vi "data表转mysql表.vi"(11 "data":string[](array[string])) -> (3 "mysqldata簇":T1 {"JCSJ" format="%<%Y/%m/%d %H:%M:%S>T"})   [LabVIEW 2016]
panel:
  out "mysql完整簇":T2 {"JCSJ" format="%<%Y/%m/%d %H:%M:%S>T"}
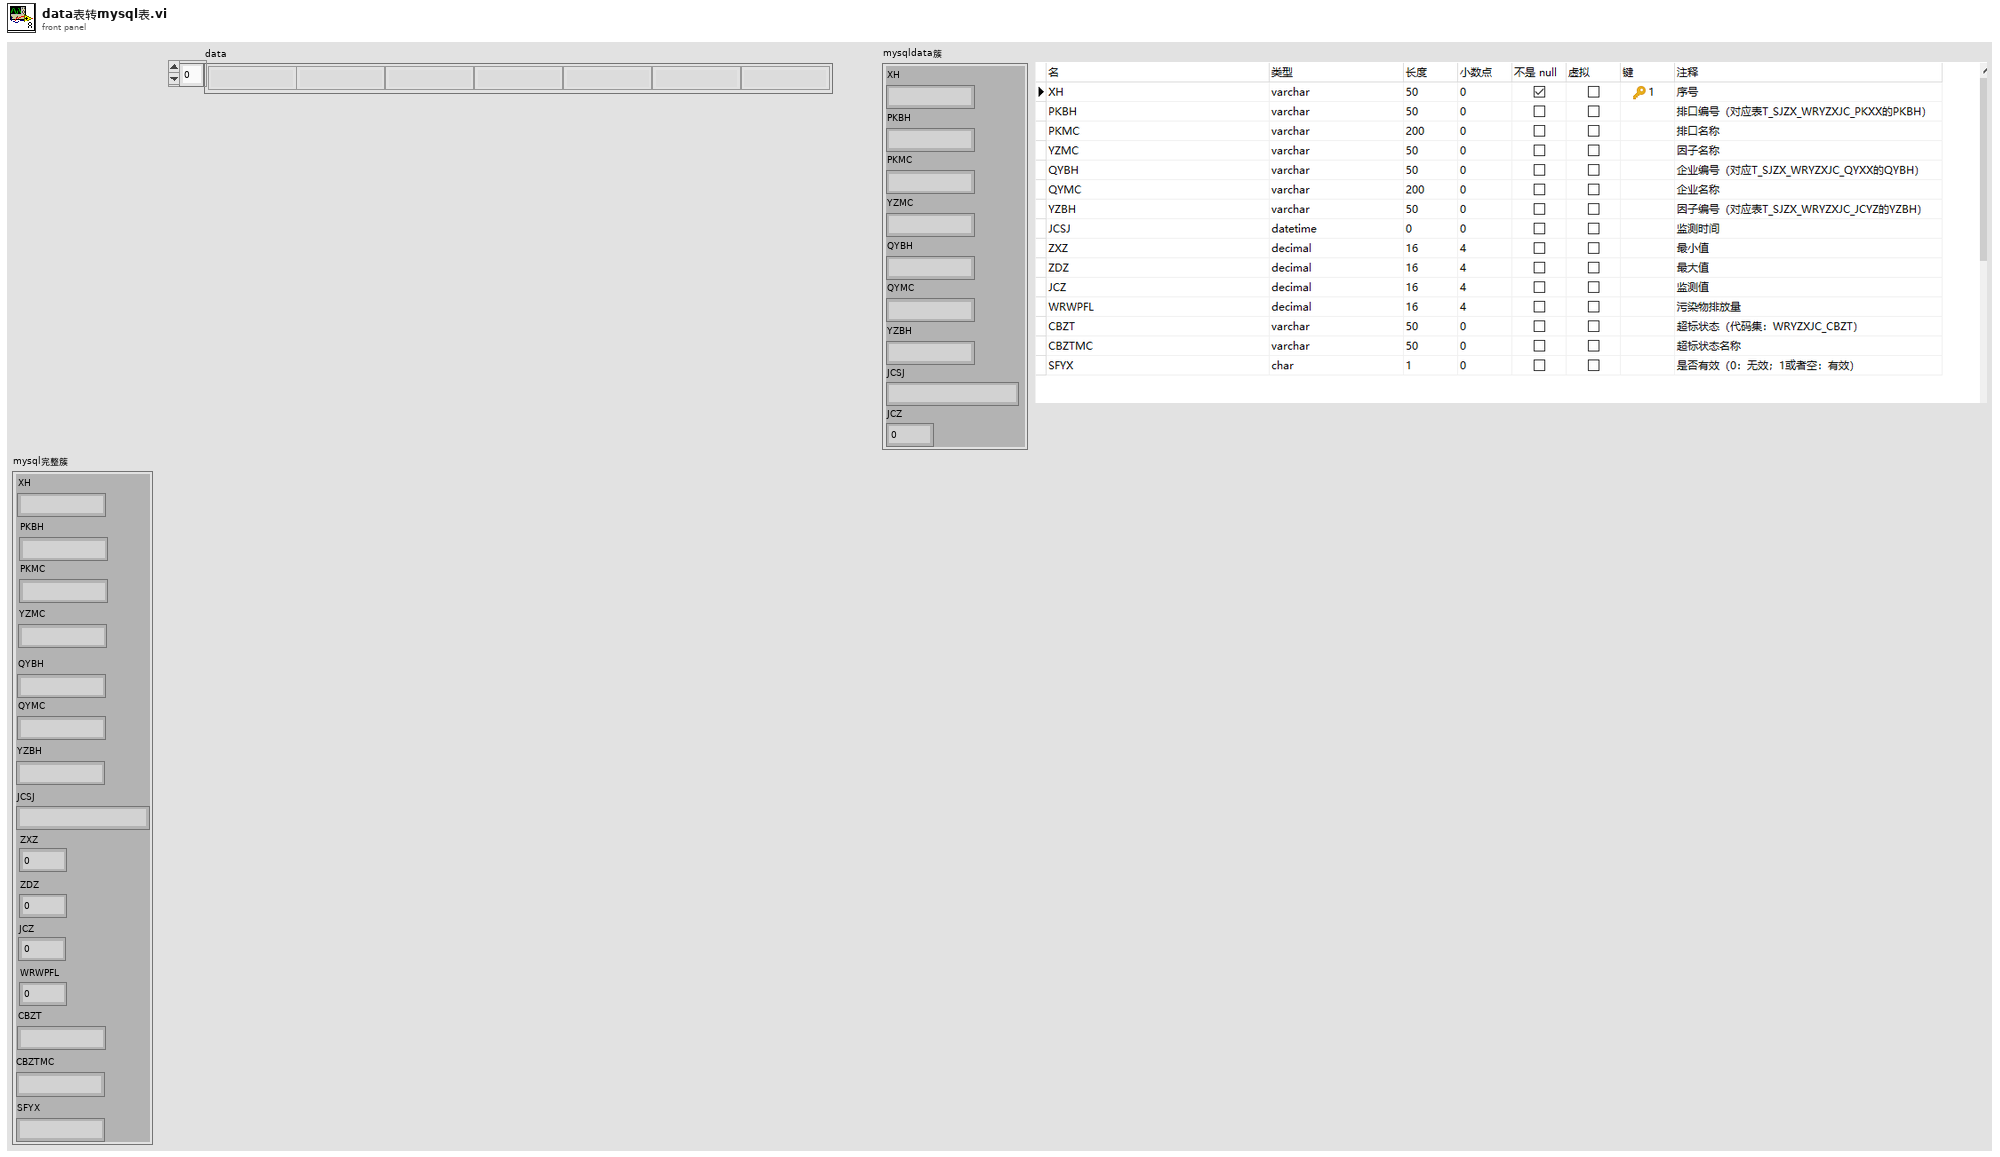
[diagram p1: front panel]
types:
  T1 = cluster{"XH":string, "PKBH":string, "PKMC":string, "YZMC":string, "QYBH":string, "QYMC":string, "YZBH":string, "JCSJ":timestamp, "JCZ":dbl}
  T2 = cluster{"XH":string, "PKBH":string, "PKMC":string, "YZMC":string, "QYBH":string, "QYMC":string, "YZBH":string, "JCSJ":timestamp, "ZXZ":dbl, "ZDZ":dbl, "JCZ":dbl, "WRWPFL":dbl, "CBZT":string, "CBZTMC":string, "SFYX":string}
  T3 = typedef "LVDateTimeRec.ctl" = cluster{"秒数的小数部分":dbl, "秒":i32, "分":i32, "时":i32, "日":i32, "月":i32, "年":i32, "天数（周）":i32, "天数（年）":i32, "DST":i32}
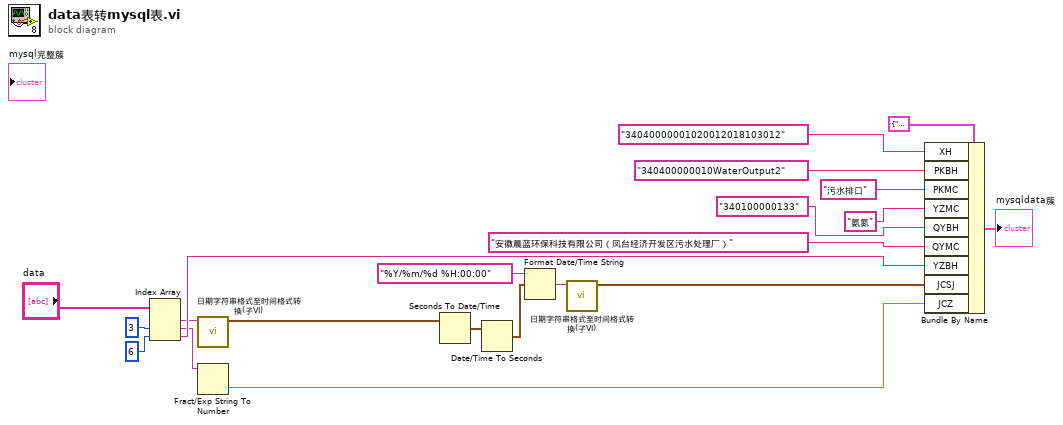
[diagram p0: block diagram]
diagram:
  n1 = Index Array(array="data", index #2=3 ("索引"), index #3=6 ("索引")) -> (element #1=w11:string, element #2=w10:string, element #3=w12:string)  [unwired: 1 in]
  n2 = call "日期字符串格式至时间格式转换(子VI).vi"("data[0]"=w11) -> ("time stamp"=w6:timestamp)  [unwired: 10 in]
  n3 = Fract/Exp String To Number(string=w10) -> (number=w9:dbl)  [unwired: 3 in, 1 out]
  n4 = Seconds To Date/Time(time stamp (now)=w6) -> (date time rec=w5:T3)  [unwired: 1 in]
  n5 = Date/Time To Seconds(2:w5) -> (0:w7:timestamp)  [unwired: 1 in]
  n6 = Format Date/Time String(time format string (%c)="%Y/%m/%d %H:00:00" ("时间格式字符串(%c)"), seconds (now)=w7) -> (date/time string=w4:string)  [unwired: 1 in]
  n7 = call "日期字符串格式至时间格式转换(子VI).vi"("data[0]"=w4) -> ("time stamp"=w3:timestamp)  [unwired: 10 in]
  n8 = Bundle By Name(cluster=T1 {"XH"="", "PKBH"="", "PKMC"="", "YZMC"="", "QYBH"="", "QYMC"="", "YZBH"="", "JCSJ"=timestamp(0 s since 1904-01-01), "JCZ"=0.0} ("mysql簇 2"), "XH"="34040000001020012018103012", "PKBH"="340400000010WaterOutput2", "PKMC"="污水排口", "YZMC"="氨氮", "QYBH"="340100000133", "QYMC"="安徽晨蓝环保科技有限公司（凤台经济开发区污水处理厂）", "YZBH"=w12, "JCSJ"=w3, "JCZ"=w9) -> (→"mysqldata簇":T1)
